vi "Alarma_Tolerancia_Frecuencia_G4.vi"(7 "ID_EQUIPO":i32=1, 11 "Señal in":sgl) -> (3 "alarm":bool)   [LabVIEW 2018]
uses:
  Global/TimerReferences.vi
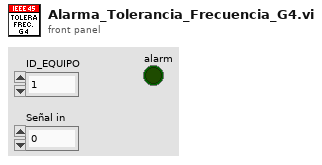
[diagram p1: front panel]
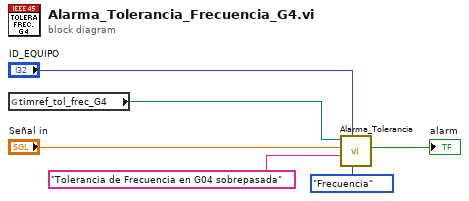
[diagram p0: block diagram]
diagram:
  n1 = global read "TimerReferences.vi" "timref_tol_frec_G4"() -> (w6:refnum<data-value>)
  n2 = call "Alarma_Tolerancia.vi"("Tipo Señal"=enum16{"Voltaje", "Frecuencia", "Voltaje AVG"}."Frecuencia", "ID_EQUIPO"="ID_EQUIPO", "Motivo Alarma"="Tolerancia de Frecuencia en G04 sobrepasada", "Señal in"="Señal in", "timref in"=w6) -> ("alarm"=→"alarm":bool)  [unwired: 6 in]
